vi "Global lettura res manuale.vi"() -> ()   [LabVIEW 2016]
panel:
  out "lettura res manuale":bool
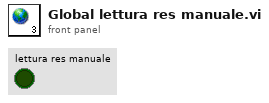
[diagram p1: front panel]
diagram:
